vi "Counter_Universal.vi"(0 "zu setzender Zählerwert":u16[](array[numeric])=[0, 0, 0, 0, 0, 0, 0, 0, 0, 0, 0, 0, 0, 0, 0, 0, 0, 0, 0, 0, 0, 0, 0, 0, 0, 0, 0, 0, 0, 0], 1 "Änderungen der Station-/Banddaten":u8[](array[numeric])=[0, 0, 0, 0, 0, 0, 0, 0, 0, 0, 0, 0, 0, 0, 0, 0, 0, 0, 0, 0], 3 "Zähler zurücksetzen":bool[](array[boolean])=[FALSE, FALSE, FALSE, FALSE, FALSE, FALSE, FALSE, FALSE, FALSE, FALSE, FALSE, FALSE, FALSE, FALSE, FALSE, FALSE, FALSE, FALSE, FALSE, FALSE, FALSE, FALSE, FALSE, FALSE, FALSE, FALSE, FALSE, FALSE, FALSE, FALSE], 4 "Zähler-Einstellung":T1(array[cluster])=[{"Index (Station/Band)"=0, "Station/Band"=enum."Station", "Bitstelle"=0, "Zählrichtung"=enum."Hochzählen"}, {"Index (Station/Band)"=0, "Station/Band"=enum."Station", "Bitstelle"=0, "Zählrichtung"=enum."Hochzählen"}, {"Index (Station/Band)"=0, "Station/Band"=enum."Station", "Bitstelle"=0, "Zählrichtung"=enum."Hochzählen"}, {"Index (Station/Band)"=0, "Station/Band"=enum."Station", "Bitstelle"=0, "Zählrichtung"=enum."Hochzählen"}, {"Index (Station/Band)"=0, "Station/Band"=enum."Station", "Bitstelle"=0, "Zählrichtung"=enum."Hochzählen"}, {"Index (Station/Band)"=0, "Station/Band"=enum."Station", "Bitstelle"=0, "Zählrichtung"=enum."Hochzählen"}, {"Index (Station/Band)"=0, "Station/Band"=enum."Station", "Bitstelle"=0, "Zählrichtung"=enum."Hochzählen"}, {"Index (Station/Band)"=0, "Station/Band"=enum."Station", "Bitstelle"=0, "Zählrichtung"=enum."Hochzählen"}, {"Index (Station/Band)"=0, "Station/Band"=enum."Station", "Bitstelle"=0, "Zählrichtung"=enum."Hochzählen"}, {"Index (Station/Band)"=0, "Station/Band"=enum."Station", "Bitstelle"=0, "Zählrichtung"=enum."Hochzählen"}, {"Index (Station/Band)"=0, "Station/Band"=enum."Station", "Bitstelle"=0, "Zählrichtung"=enum."Hochzählen"}, {"Index (Station/Band)"=0, "Station/Band"=enum."Station", "Bitstelle"=0, "Zählrichtung"=enum."Hochzählen"}, {"Index (Station/Band)"=0, "Station/Band"=enum."Station", "Bitstelle"=0, "Zählrichtung"=enum."Hochzählen"}, {"Index (Station/Band)"=0, "Station/Band"=enum."Station", "Bitstelle"=0, "Zählrichtung"=enum."Hochzählen"}, {"Index (Station/Band)"=0, "Station/Band"=enum."Station", "Bitstelle"=0, "Zählrichtung"=enum."Hochzählen"}, {"Index (Station/Band)"=0, "Station/Band"=enum."Station", "Bitstelle"=0, "Zählrichtung"=enum."Hochzählen"}, {"Index (Station/Band)"=0, "Station/Band"=enum."Station", "Bitstelle"=0, "Zählrichtung"=enum."Hochzählen"}, {"Index (Station/Band)"=0, "Station/Band"=enum."Station", "Bitstelle"=0, "Zählrichtung"=enum."Hochzählen"}, {"Index (Station/Band)"=0, "Station/Band"=enum."Station", "Bitstelle"=0, "Zählrichtung"=enum."Hochzählen"}, {"Index (Station/Band)"=0, "Station/Band"=enum."Station", "Bitstelle"=0, "Zählrichtung"=enum."Hochzählen"}, {"Index (Station/Band)"=0, "Station/Band"=enum."Station", "Bitstelle"=0, "Zählrichtung"=enum."Hochzählen"}, {"Index (Station/Band)"=0, "Station/Band"=enum."Station", "Bitstelle"=0, "Zählrichtung"=enum."Hochzählen"}, {"Index (Station/Band)"=0, "Station/Band"=enum."Station", "Bitstelle"=0, "Zählrichtung"=enum."Hochzählen"}, {"Index (Station/Band)"=0, "Station/Band"=enum."Station", "Bitstelle"=0, "Zählrichtung"=enum."Hochzählen"}, {"Index (Station/Band)"=0, "Station/Band"=enum."Station", "Bitstelle"=0, "Zählrichtung"=enum."Hochzählen"}, {"Index (Station/Band)"=0, "Station/Band"=enum."Station", "Bitstelle"=0, "Zählrichtung"=enum."Hochzählen"}, {"Index (Station/Band)"=0, "Station/Band"=enum."Station", "Bitstelle"=0, "Zählrichtung"=enum."Hochzählen"}, {"Index (Station/Band)"=0, "Station/Band"=enum."Station", "Bitstelle"=0, "Zählrichtung"=enum."Hochzählen"}, {"Index (Station/Band)"=0, "Station/Band"=enum."Station", "Bitstelle"=0, "Zählrichtung"=enum."Hochzählen"}, {"Index (Station/Band)"=0, "Station/Band"=enum."Station", "Bitstelle"=0, "Zählrichtung"=enum."Hochzählen"}]) -> (7 "Counter":u16[](array[numeric]))   [LabVIEW 2013]
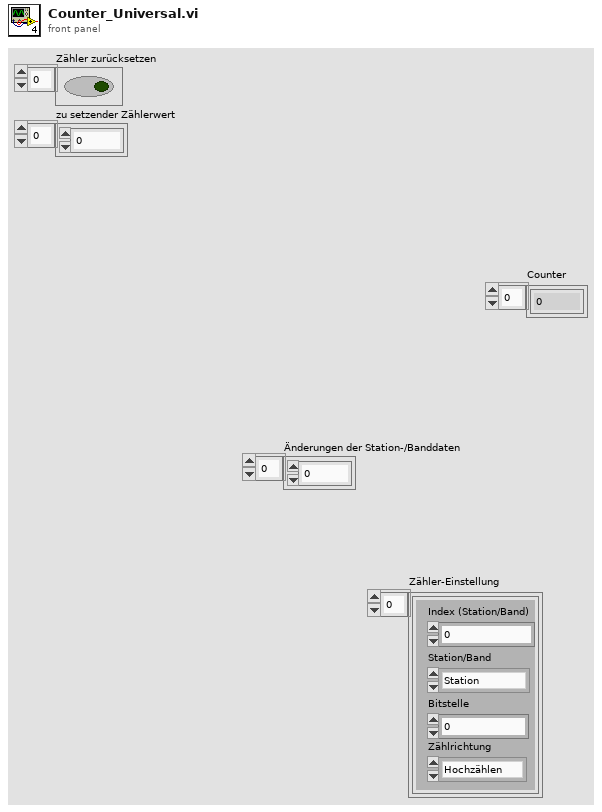
[diagram p1: front panel]
types:
  T1 = cluster{"Index (Station/Band)":u8, "Station/Band":enum16{"Station", "Band"}, "Bitstelle":u8, "Zählrichtung":enum16{"Hochzählen", "Runterzählen"}}[]
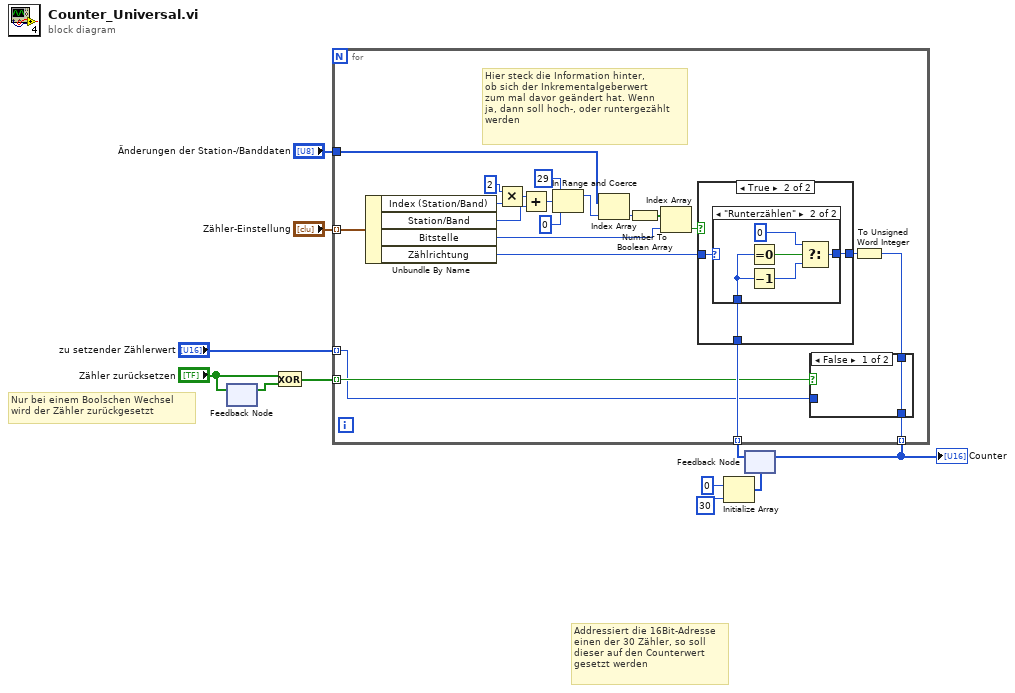
[diagram p0: block diagram]
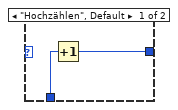
[diagram p4: hidden frame]
diagram:
  # "Nur bei einem Boolschen Wechsel \nwird der Zähler zurückgesetzt"
  # "Addressiert die 16Bit-Adresse\neinen der 30 Zähler, so soll \ndieser auf den Counterwert\ngesetzt werden"
  n1 = feedback-in #1("Zähler zurücksetzen") -> ()
  n2 = feedback #1() -> (w4:bool[])  [unwired: 1 in]
  n3 = Exclusive Or(1:w4, 2:"Zähler zurücksetzen") -> (0:w2:bool[])
  n4 = Initialize Array(u16 0, 30 ("Dimension")) -> (w7:u16[])
  n5 = feedback #2(w7) -> (w11:u16[])
  n6 = for {
    tunnel: "Änderungen der Station-/Banddaten" -> [w32]
    tunnel: [w14] -> w5 mode=indexing
    tunnel: w11 -> [w25] mode=indexing
    tunnel: "Zähler-Einstellung" -> [w29] mode=indexing
    tunnel: w2 -> [w13] mode=indexing
    tunnel: "zu setzender Zählerwert" -> [w12] mode=indexing
    # "Hier steck die Information hinter,\nob sich der Inkrementalgeberwert\nzum mal davor geändert hat. Wenn\nja, dann soll hoch-, oder runtergezählt\nwerden"
    n7 = Unbundle By Name(w29) -> ("Index (Station/Band)"=w24:u8, "Station/Band"=w22:enum16{"Station", "Band"}, "Bitstelle"=w27:u8, "Zählrichtung"=w26:enum16{"Hochzählen", "Runterzählen"})
    n8 = Multiply(x=u8 2, y=w24) -> (x*y=w21:u8)
    n9 = Add(x=w21, y=w22) -> (x+y=w19:u16)
    n10 = In Range and Coerce(upper limit=u16 29 ("Obergrenze"), x=w19, lower limit=u16 0 ("Untergrenze")) -> (coerced(x)=w20:u16)  [unwired: 1 out]
    n11 = Index Array(array=w32, index=w20) -> (element=w31:u8)
    n12 = Number To Boolean Array(number=w31) -> (Boolean array=w30:bool[])
    n13 = Index Array(array=w30, index=w27) -> (element=w28:bool)
    n14 = case shown="True" w28 {
      tunnel: w26 -> [_ w38]
      tunnel: w25 -> [w35 w37]
      tunnel: [w35 w36] -> w16
      frame False {
      }
      frame True {
        n15 = case shown="\"Runterzählen\"" w38 {
          tunnel: w37 -> [w39 w41]
          tunnel: [w40 w45] -> w36
          frame "Hochzählen", Default {
            n16 = Increment(x=w39) -> (x+1=w40:u16)
          }
          frame "Runterzählen" {
            n17 = Equal To 0?(x=w41) -> (x = 0?=w42:bool)
            n18 = Decrement(x=w41) -> (x-1=w43:u16)
            n19 = Select(t=u16 0, s=w42, f=w43) -> (s? t:f=w45:u16)
          }
        }
      }
    }
    n20 = To Unsigned Word Integer(number=w16) -> (unsigned 16bit integer=w15:u16)
    n21 = case shown="False" w13 {
      tunnel: w15 -> [w33 _]
      tunnel: [w33 w34] -> w14
      tunnel: w12 -> [_ w34]
      frame False {
      }
      frame True {
      }
    }
  }
  "Counter" <- w5
  n22 = feedback-in #2(w5) -> ()
